vi "FIR Narrowband Coefficients.vi"(0 "sampling freq: fs":dbl=1.0 min=0.0 format="%0.2f", 1 "ripple: rp":dbl=0.01 min=0.0 format="%0.4f", 2 "passband: fpass":dbl=0.01 min=0.0 format="%0.4f", 3 "stopband: fstop":dbl=0.02 min=0.0 format="%0.4f", 4 "attenuation (db): Ar":dbl=60.0 min=0.0 format="%0.1f", 5 "center freq: fc":dbl=0.2 min=0.0 format="%0.4f", 8 "filter type":T2) -> (6 "IFIR Coefficients":T1 {"Image Suppressor" format="%.2e"; "Model Filter" format="%.2e"}, 7 "error":i32)   [LabVIEW 2017, in "NI_AALBase.lvlib"]
doc: "Generates a set of filter coefficients to implement a digital interpolated FIR (IFIR) filter."
uses:
  <vilib>/Analysis/NI_AALBase.lvlib
  <vilib>/Analysis/3filter.llb/Filter Passband Type.ctl
  <resource>/lvanlys.dll
panel:
  # "FIR Narrowband\n Coefficients"
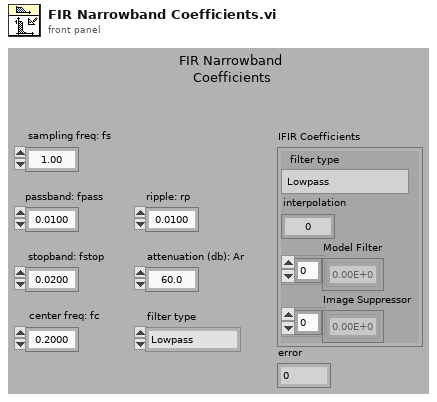
[diagram p1: front panel]
types:
  T1 = cluster{"filter type":enum32{"Lowpass", "Highpass", "Bandpass", "Bandstop", "Wideband-Lowpass", "Wideband-Highpass"}, "interpolation":i32, "Model Filter":dbl[], "Image Suppressor":dbl[]}
  T2 = typedef "NI_AALBase.lvlib/Filter Passband Type.ctl" = enum32{"Lowpass", "Highpass", "Bandpass", "Bandstop"}
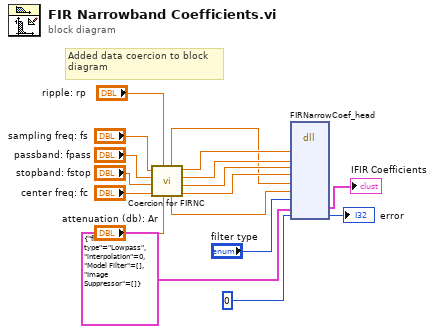
[diagram p0: block diagram]
diagram:
  # "Added data coercion to block\ndiagram"
  n1 = call <vilib>:"Coercion for FIRNC.vi"("attenuation (db): Ar"="attenuation (db): Ar", "ripple: rp"="ripple: rp", "center freq: fc"="center freq: fc", "stopband: fstop"="stopband: fstop", "passband: fpass"="passband: fpass", "sampling freq: fs"="sampling freq: fs") -> ("center freq: fc"=w5:dbl, "stopband: fstop"=w6:dbl, "passband: fpass"=w7:dbl, "sampling freq: fs"=w8:dbl, "attenuation (db): Ar"=w4:dbl, "ripple: rp"=w3:dbl)
  n2 = dll-call lib="e:/builds/penguin/labview/branches/2017/dev/dist/resource/lvanlys.*" fn="FIRNarrowCoef_head"("sampling freq: fs"=w8, "passband: fpass"=w7, "stopband: fstop"=w6, "center freq: fc"=w5, "ripple: rp"=w3, "attenuation (db): Ar"=w4, "filter type"="filter type", "IFIR Coefficients"=T1 {"filter type"=enum."Lowpass", "interpolation"=0, "Model Filter"=[], "Image Suppressor"=[]}, "output param"=0) -> ("IFIR Coefficients"=→"IFIR Coefficients":T1, "output param"=→"error":i32)  [unwired: 10 in, 3 out]
